vi "Create Channel Properties Cluster.vi"(8 "error in":errorcluster, 9 "Channel Type":string, 10 "Settings Cluster Path":path, 11 "Clust Refnum":refnum<vi>) -> (0 "error out":errorcluster, 3 "Clust Refnum":refnum<vi>)   [LabVIEW 2026, in "Plugin XML Parser.lvlib"]
uses:
  Plugin XML Parser.lvlib
  <vilib>/Utility/miscctls.llb/LVPointTypeDef.ctl
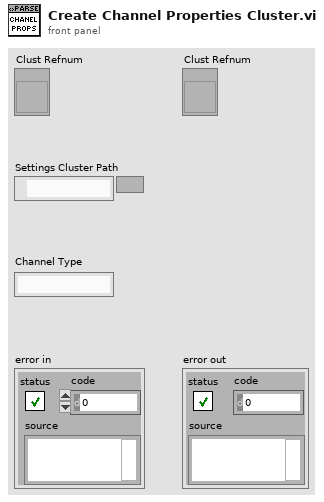
[diagram p1: front panel]
types:
  T1 = enum32{"not a control VI", "control", "typedef", "strict typedef"}
  T2 = enum32{"invalid VI type", "Standard VI", "Control VI", "Global VI", "Polymorphic VI", "Configuration VI", "SubSystem", "Facade VI", "Method VI", "Statechart Diagram VI"}
  T3 = typedef "LVPointTypeDef.ctl" = cluster{"Horizontal":i16, "Vertical":i16}
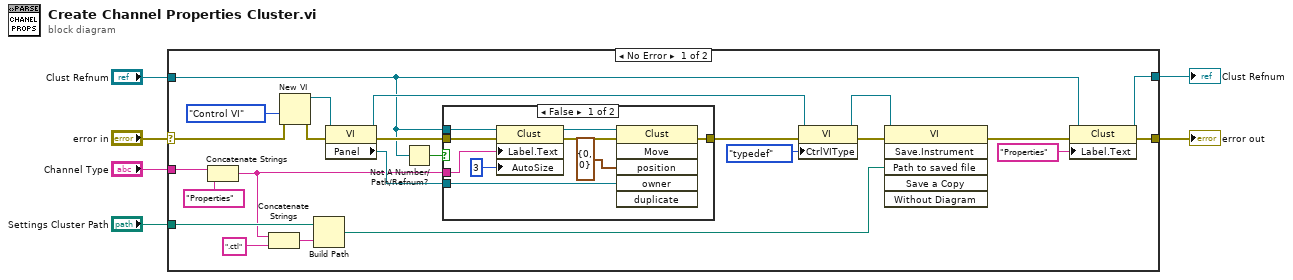
[diagram p0: block diagram]
diagram:
  n1 = case shown="No Error" "error in" {
    selector: "error in" -> [w29 w42]
    tunnel: "Clust Refnum" -> [w8 w41]
    tunnel: [w10 w41] -> w3
    tunnel: [w24 w42] -> w6
    tunnel: "Settings Cluster Path" -> [w23 _]
    tunnel: "Channel Type" -> [w20 _]
    frame No Error {
      n2 = Concatenate Strings(w20, "Properties" ("string")) -> (w7:string)
      n3 = Concatenate Strings(w7, ".ctl" ("string")) -> (w16:string)
      n4 = New VI(8:w29, 9:T2."Control VI" ("vi type (standard vi)")) -> (0:w28:errorcluster, 3:w13:refnum<vi>)  [unwired: 5 in]
      n5 = Build Path(base path=w23, name or relative path=w16) -> (appended path=w22:path)
      n6 = property class="VI"(reference=w13, error in=w28) -> (reference out=w12:refnum<vi>, error out=w25:errorcluster, "Panel"=w11:refnum<vi>)
      n7 = Not A Number/Path/Refnum?(number/path/refnum=w8) -> (NaN/Path/Refnum?=w14:bool)
      n8 = case shown="False" w14 {
        tunnel: [w39 w40] -> w27
        tunnel: w25 -> [w38 w40]
        tunnel: w8 -> [w34 _]
        tunnel: w11 -> [w36 _]
        tunnel: w7 -> [w32 _]
        frame False {
          n9 = property class="Clust"(reference=w34, error in=w38, "Label.Text"=w32, "AutoSize"=u32 3 ("Auto Sizing")) -> (reference out=w33:refnum<vi>, error out=w37:errorcluster)
          n10 = invoke class="Clust" method="Move"(reference=w33, error in=w37, "position"=T3 {"Horizontal"=0, "Vertical"=0} ("location"), "owner"=w36) -> (error out=w39:errorcluster)  [unwired: 2 in, 5 out]
        }
        frame True {
        }
      }
      n11 = property class="VI"(reference=w12, error in=w27, "CtrlVIType"=T1."typedef" ("Control VI Type")) -> (reference out=w17:refnum<vi>, error out=w26:errorcluster)
      n12 = invoke class="VI" method="Save.Instrument"(reference=w17, error in=w26, "Path to saved file"=w22) -> (error out=w30:errorcluster)  [unwired: 3 in, 5 out]
      n13 = property class="Clust"(reference=w8, error in=w30, "Label.Text"="Properties") -> (reference out=w10:refnum<vi>, error out=w24:errorcluster)
    }
    frame Error {
    }
  }
  "error out" <- w6
  "Clust Refnum" <- w3
